vi "ROS2 Start.vi"() -> (1 "reader error":errorcluster[](array[cluster]), 2 "Writer":u64[](array[numeric]), 3 "writer error":errorcluster[](array[cluster]), 4 "Reader":u64[](array[numeric]))   [LabVIEW 2021]
uses:
  <vilib>/RTI DDS Toolkit/Types/RTI DDS Advanced Writer Configuration.ctl
  <vilib>/RTI DDS Toolkit/Types/RTI DDS Advanced Reader Configuration.ctl
  <vilib>/RTI DDS Toolkit/VIs/AdvancedCreateWriter_NumI32.vi
  <vilib>/RTI DDS Toolkit/VIs/AdvancedCreateReader_NumI32.vi
  <vilib>/RTI DDS Toolkit/Library/LVDDS_library.lvlib
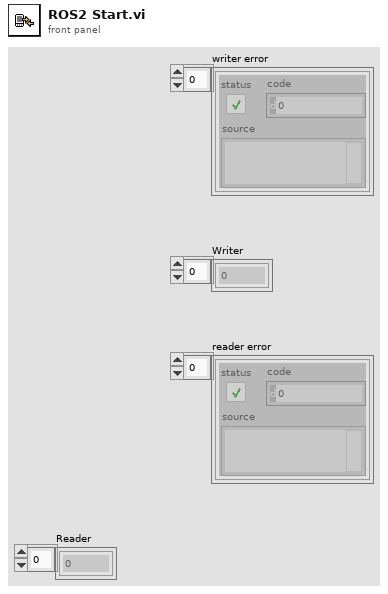
[diagram p1: front panel]
types:
  T1 = typedef "LVDDS_library.lvlib/RTI DDS Advanced Reader Configuration.ctl" = cluster{"typeName":string, "keyName":string, "domainParticipantQoSProfile":string, "dataReaderQoSProfile":string, "forceArrayMapping?":bool, "forceExclusiveReader?":bool, "forceRead? (only ExclusiveReader)":bool, "forceUnboundedString?":bool}
  T2 = typedef "LVDDS_library.lvlib/RTI DDS Advanced Writer Configuration.ctl" = cluster{"typeName":string, "keyName":string, "domainParticipantQoSProfile":string, "dataWriterQoSProfile":string, "forceArrayMapping?":bool, "forceUnboundedString?":bool}
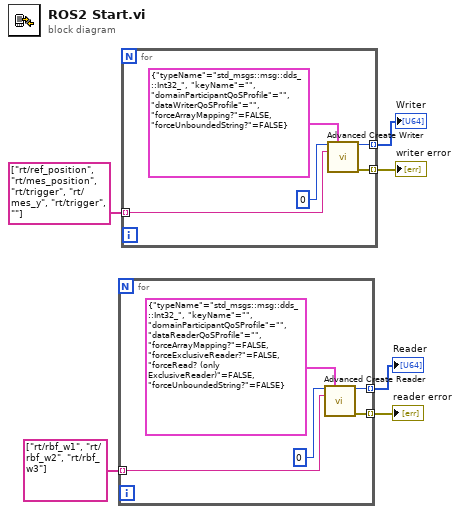
[diagram p0: block diagram]
diagram:
  n1 = for {
    tunnel: string[] ["rt/rbf_w1", "rt/rbf_w2", "rt/rbf_w3"] ("Topic Name") -> [w9] mode=indexing
    tunnel: [w8] -> w3 mode=indexing
    tunnel: [w7] -> w4 mode=indexing
    n2 = call-poly <vilib>:"Advanced Create Reader.vi"("Domain Id"=u32 0, "Advanced Reader Configuration"=T1 {"typeName"="std_msgs::msg::dds_::Int32_", "keyName"="", "domainParticipantQoSProfile"="", "dataReaderQoSProfile"="", "forceArrayMapping?"=FALSE, "forceExclusiveReader?"=FALSE, "forceRead? (only ExclusiveReader)"=FALSE, "forceUnboundedString?"=FALSE} ("Advanced Reader Configuration 3"), "Topic Name"=w9) -> ("DDS Object Ref"=w8:u64, "error out"=w7:errorcluster)  [unwired: 11 in]
  }
  "reader error" <- w4
  "Reader" <- w3
  n3 = for {
    tunnel: [w16] -> w2 mode=indexing
    tunnel: [w15] -> w1 mode=indexing
    tunnel: string[] ["rt/ref_position", "rt/mes_position", "rt/trigger", "rt/mes_y", "rt/trigger", ""] ("Topic Name") -> [w12] mode=indexing
    n4 = call-poly <vilib>:"Advanced Create Writer.vi"("Domain Id"=u32 0, "Advanced Writer Configuration"=T2 {"typeName"="std_msgs::msg::dds_::Int32_", "keyName"="", "domainParticipantQoSProfile"="", "dataWriterQoSProfile"="", "forceArrayMapping?"=FALSE, "forceUnboundedString?"=FALSE}, "Topic Name"=w12) -> ("DDS Object Ref"=w15:u64, "error out"=w16:errorcluster)  [unwired: 11 in]
  }
  "writer error" <- w2
  "Writer" <- w1
